vi "Get lvclass Ref in Active Project.vi"(8 "error in (no error)":errorcluster, 11 "File":path) -> (0 "error out":errorcluster, 3 "LVClassLibrary out":refnum<vi>)   [LabVIEW 2020, in "Mock Class Updater.lvclass"]
uses:
  Mock Class Updater.lvclass
  Mock Class Updater.lvclass/Mock Class Updater.ctl
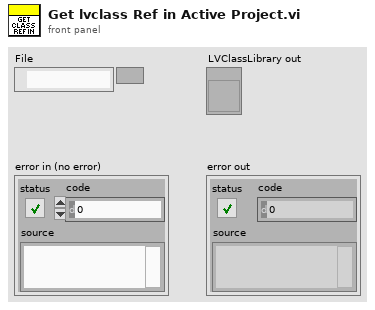
[diagram p1: front panel]
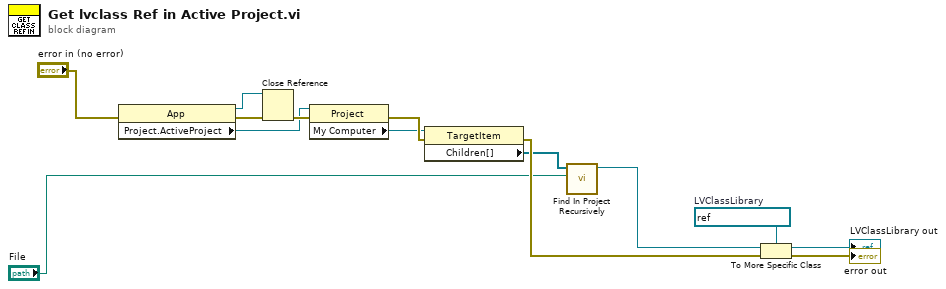
[diagram p0: block diagram]
diagram:
  w9 = refnum<vi> refnum  # LVClassLibrary
  n1 = property class="App"(error in="error in (no error)") -> (reference out=w6:refnum<vi>, error out=w4:errorcluster, "Project.ActiveProject"=w3:refnum<vi>)  [unwired: 1 in]
  n2 = Close Reference(reference=w6, error in (no error)=w4) -> (error out=w5:errorcluster)
  n3 = property class="Project"(reference=w3, error in=w5) -> (error out=w12:errorcluster, "My Computer"=w7:refnum<vi>)  [unwired: 1 out]
  n4 = property class="TargetItem"(reference=w7, error in=w12) -> (error out=w11:errorcluster, "Children[]"=w2:refnum<vi>[])  [unwired: 1 out]
  n5 = call "Find In Project Recursively.vi"("File"="File", "Project Items"=w2) -> ("ProjectItem out"=w14:refnum<vi>)  [unwired: 9 in]
  n6 = To More Specific Class(target class=w9, reference=w14, error in=w11) -> (specific class reference=→"LVClassLibrary out":refnum<vi>, error out=→"error out":errorcluster)
